vi "KE2606 Measuring.vi"(11 "VISA":refnum<visa-resource-name>) -> ()   [LabVIEW 2017]
doc: "This example shows how to configure the source and take a measurement."
uses:
  Channel.ctl
  Mesuring State.ctl
  <instrlib>/Keithley 2600 Series/Public/Channel.ctl
  <instrlib>/Keithley 2600 Series/Keithley 2600 Series.lvlib
panel:
  in  "Channel (Channel A)":T1
  in  "Voltage step, V":dbl=0.05
  in  "Voltage stop, V":dbl=2.0
  in  "Voltage start, V":dbl
  in  "Current limit, A":dbl=1.0
  in  "Channel":T2
  out "Measured current, A":dbl
  out "Sourced voltage, V":dbl
  out "I/V Curve":cluster{"X":dbl, "Y":dbl}[](graph) caption="XY Graph - Light"
  out "State":T3
  in  "Stop Button":bool
  in  "Start Button":bool
  in  "Exit Button":bool
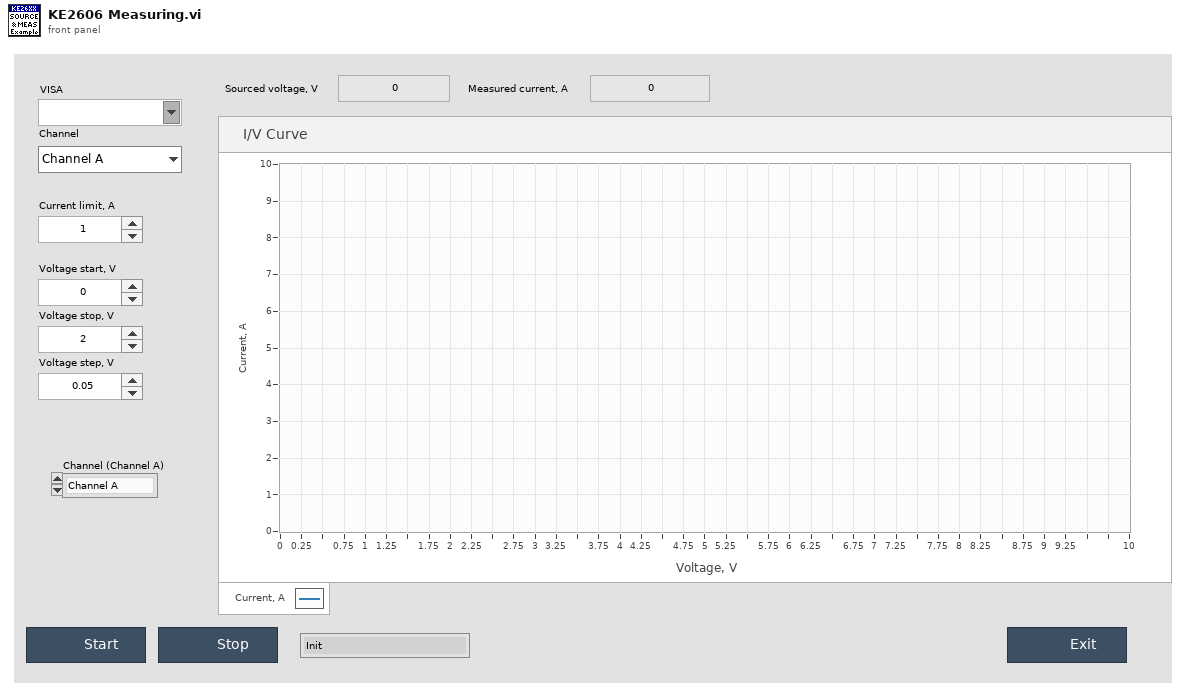
[diagram p1: front panel]
types:
  T1 = typedef "Keithley 2600 Series.lvlib/Channel.ctl" = enum32{"Channel A", "Channel B"}
  T2 = typedef "Channel.ctl" = enum32{"Channel A", "Channel B"}
  T3 = typedef "Mesuring State.ctl" = enum16{"Init", "Start", "Stop", "Nothing", "Exit"}
  T4 = enum32{"Current", "Voltage", "IV", "Resistance", "Power"}
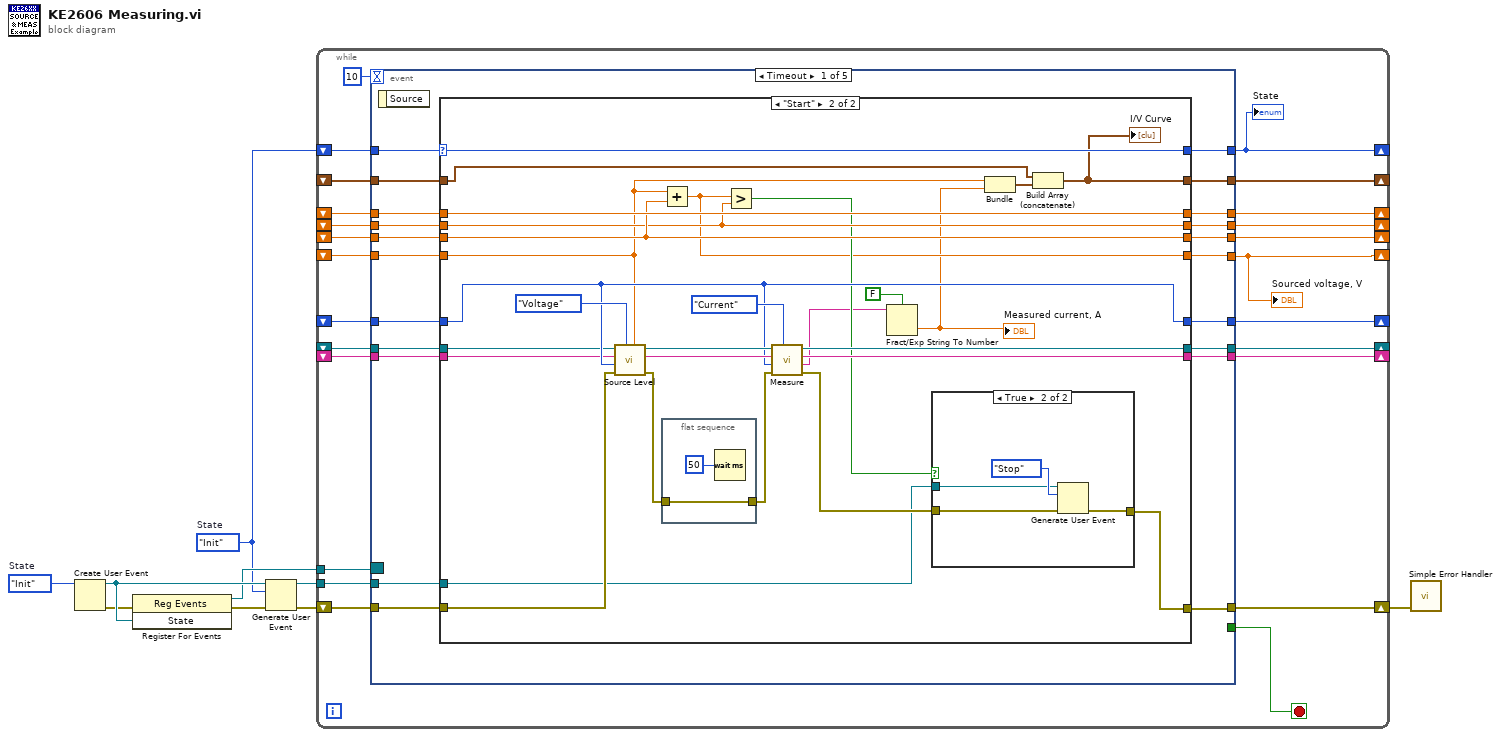
[diagram p0: block diagram]
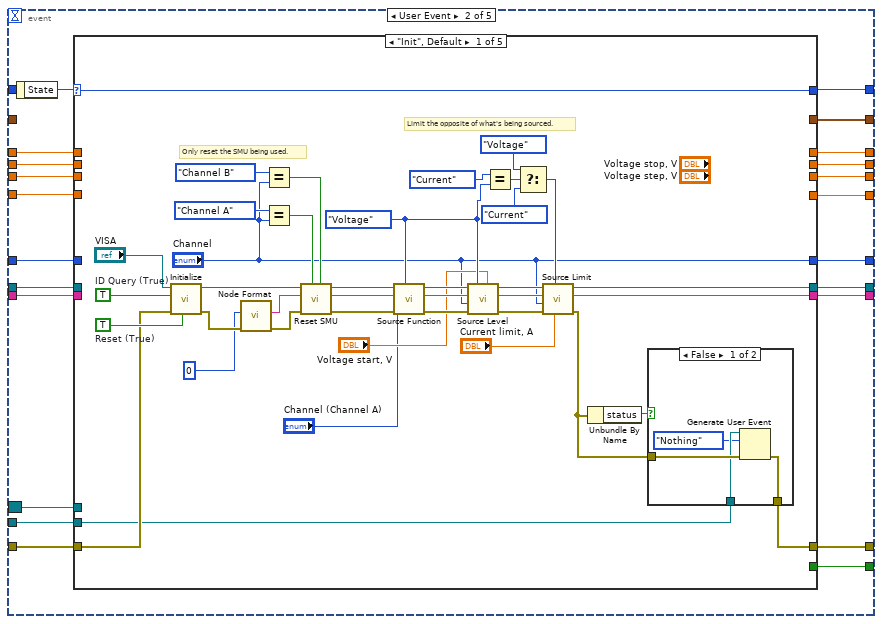
[diagram p4: hidden frame]
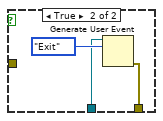
[diagram p5: hidden frame]
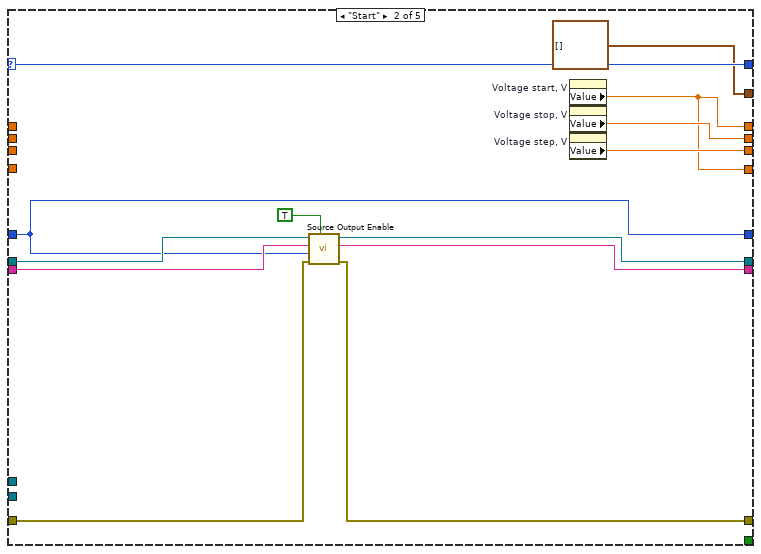
[diagram p6: hidden frame]
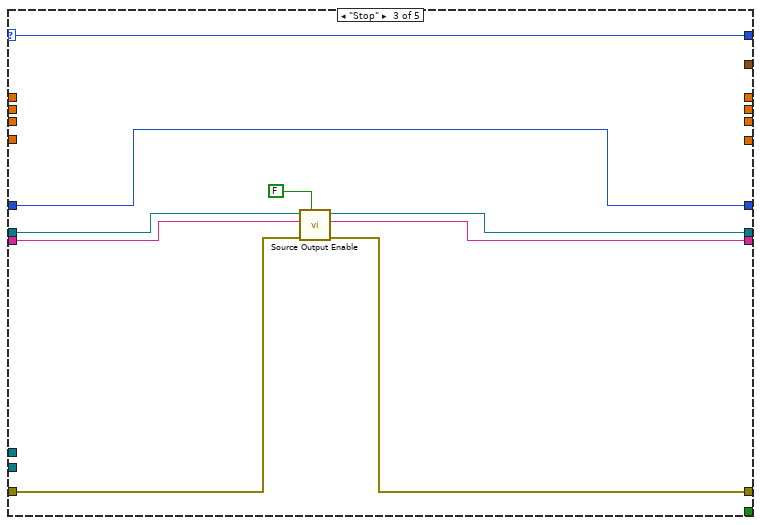
[diagram p7: hidden frame]
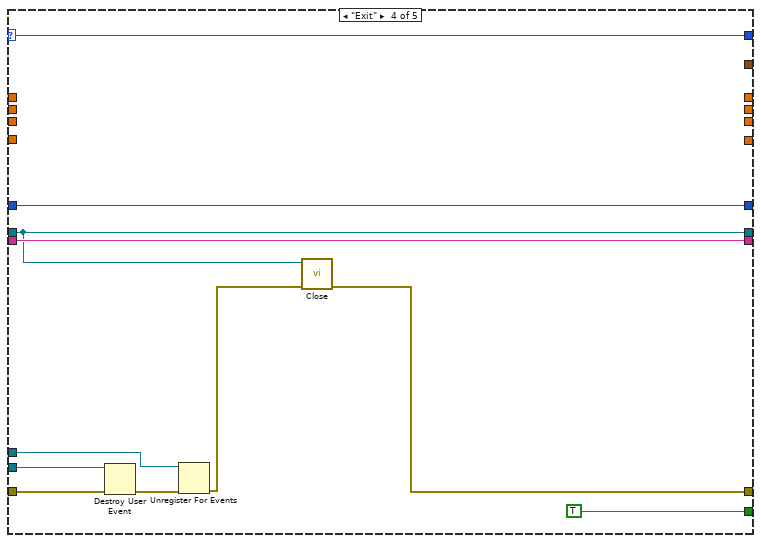
[diagram p8: hidden frame]
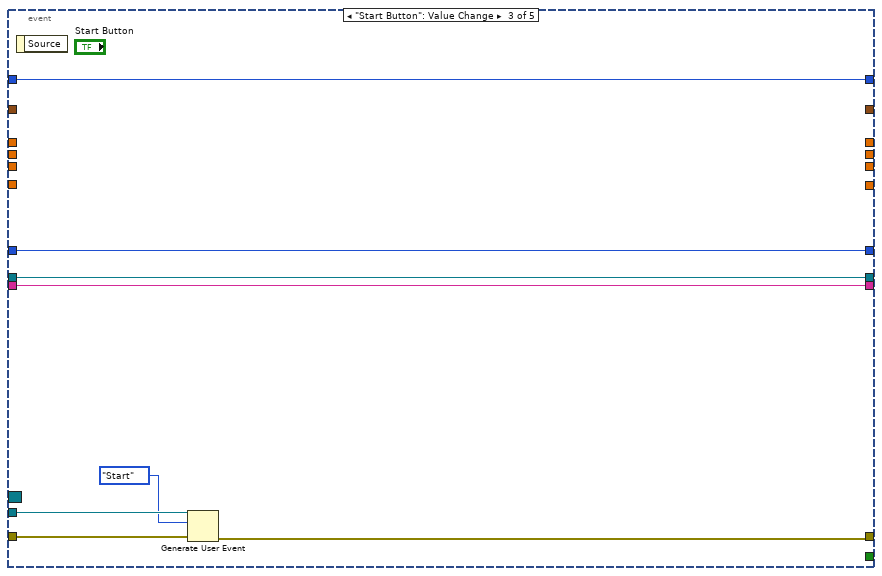
[diagram p10: hidden frame]
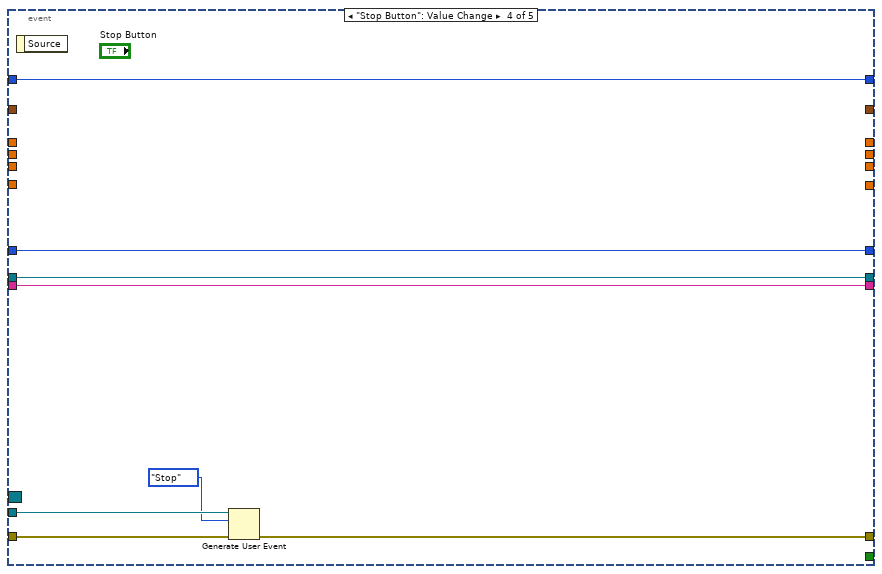
[diagram p11: hidden frame]
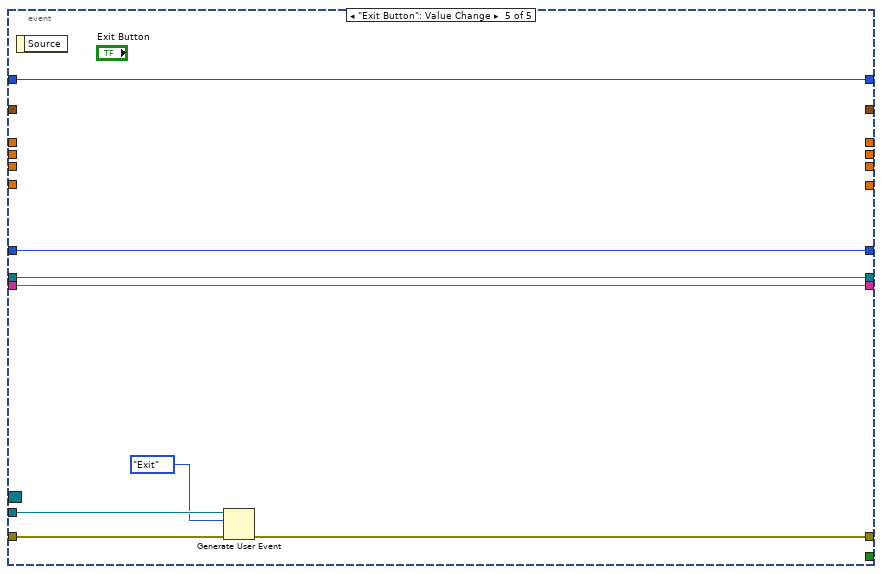
[diagram p12: hidden frame]
diagram:
  w1 = Mesuring_State."Init"  # State
  w3 = Mesuring_State."Init"  # State
  n1 = Create User Event(user event datatype=w3) -> (user event=w9:refnum<user-event>, error out=w7:errorcluster)  [unwired: 1 in]
  n2 = register-events(error in=w7, w9) -> (reference out=w6:refnum<event-registration>, error out=w8:errorcluster)  [unwired: 1 in]
  n3 = Generate User Event(user event=w9, event data cluster=w1, error in=w8) -> (user event out=w5:refnum<user-event>, error out=w4:errorcluster)  [unwired: 1 in]
  n4 = while {
    tunnel: w6 -> [w31]
    tunnel: w5 -> [w32]
    shift-right: [w30] -> w2
    shift-left: w4 -> [w33]
    shift-right: [w29] -> _
    shift-left: _ -> [w25]
    shift-right: [w28] -> _
    shift-left: _ -> [w24]
    shift-right: [w27] -> _
    shift-left: _ -> [w26]
    shift-right: [w23] -> _
    shift-left: w1 -> [w22]
    shift-right: [w19] -> _
    shift-left: _ -> [w15]
    shift-right: [w18] -> _
    shift-left: _ -> [w14]
    shift-right: [w17] -> _
    shift-left: _ -> [w16]
    shift-right: [w12] -> _
    shift-left: _ -> [w13]
    shift-right: [w11] -> _
    shift-left: _ -> [w10]
    stop <- w20 stop-if-true
    n5 = event shown="[0] Timeout" {
      selector: w31 -> [_ w110 _ _ _]
      dyn-events: _ -> [_ _ _ _ _]
      timeout: 10 -> [_ _ _ _ _]
      tunnel: w33 -> [w46 w119 w208 w217 w224]
      tunnel: w32 -> [w36 w120 w209 w215 w225]
      tunnel: [w45 w118 w207 w216 w222] -> w30
      tunnel: [w49 w117 w211 w219 w227] -> w29
      tunnel: [w47 w116 w210 w218 w226] -> w28
      tunnel: [w51 w115 w212 w220 w228] -> w27
      tunnel: w26 -> [w52 w114 w212 w220 w228]
      tunnel: w25 -> [w50 w113 w211 w219 w227]
      tunnel: w24 -> [w48 w112 w210 w218 w226]
      tunnel: [w53 w111 w213 w221 w229] -> w23
      tunnel: w22 -> [w54 _ w213 w221 w229]
      tunnel: [_ w109 _ _ _] -> w20
      tunnel: [w39 w108 _ _ _] -> w19
      tunnel: [w38 w107 _ _ _] -> w18
      tunnel: [w43 w106 _ _ _] -> w17
      tunnel: w16 -> [w44 w105 _ _ _]
      tunnel: w15 -> [w42 w104 _ _ _]
      tunnel: w14 -> [w41 w103 _ _ _]
      tunnel: [w37 w102 _ _ _] -> w12
      tunnel: w13 -> [w40 w101 _ _ _]
      tunnel: [w35 w100 _ _ _] -> w11
      tunnel: w10 -> [w34 _ _ _ _]
      event Timeout {
        n6 = event-data() -> ()  [unwired: 1 in, 1 out]
        n7 = case shown="\"Start\"" w54 {
          selector: w54 -> [w64 w92]
          tunnel: [w64 w92] -> w53
          tunnel: [w63 w85] -> w51
          tunnel: w52 -> [w63 w85]
          tunnel: w50 -> [w62 w84]
          tunnel: [w62 w89] -> w49
          tunnel: w48 -> [w61 w83]
          tunnel: [w61 w90] -> w47
          tunnel: w46 -> [w60 w82]
          tunnel: [w60 w76] -> w45
          tunnel: [w59 w81] -> w43
          tunnel: w44 -> [w59 w81]
          tunnel: w42 -> [w58 w79]
          tunnel: w41 -> [w57 w80]
          tunnel: w40 -> [w56 w71]
          tunnel: [w58 w79] -> w39
          tunnel: [w57 w80] -> w38
          tunnel: [w56 w75] -> w37
          tunnel: w36 -> [_ w74]
          tunnel: [w55 w67] -> w35
          tunnel: w34 -> [w55 w68]
          frame Default {
          }
          frame "Start" {
            n8 = call <instrlib>:"Source Level.vi"("Level (0.000)"=w71, "Function (Current)"=enum32{"Current", "Voltage"}."Voltage", "error in (no error)"=w82, "Channel (Channel A)"=w85, "Node In"=w83, "VISA resource name"=w84) -> ("error out"=w66:errorcluster, "Node Out"=w87:string, "VISA resource name out"=w86:refnum<visa-resource-name>)  [unwired: 3 out]
            n9 = Add(x=w71, y=w80) -> (x+y=w75:dbl)
            n10 = flat-sequence {
              tunnel: w66 -> [w94]
              tunnel: [w94] -> w65
              frame #0 {
                n11 = Wait (ms)(milliseconds to wait=u32 50) -> ()  [unwired: 1 out]
              }
            }
            n12 = Greater?(x=w75, y=w79) -> (0:w78:bool)
            n13 = call <instrlib>:"Measure.vi"("Function (Current)"=T4."Current", "error in (no error)"=w65, "Channel (Channel A)"=w85, "Node In"=w87, "VISA resource name"=w86) -> ("error out"=w77:errorcluster, "Output"=w73:string, "Node Out"=w90:string, "VISA resource name out"=w89:refnum<visa-resource-name>)  [unwired: 2 in, 1 out]
            n14 = Fract/Exp String To Number(use system decimal point (T)=FALSE, string=w73) -> (number=w70:dbl)  [unwired: 2 in, 1 out]
            "Measured current, A" <- w70
            n15 = case shown="True" w78 {
              tunnel: w77 -> [w95 w98]
              tunnel: [w95 w97] -> w76
              tunnel: w74 -> [_ w96]
              frame False {
              }
              frame True {
                n16 = Generate User Event(user event=w96, event data cluster=Mesuring_State."Stop" ("event data"), error in=w98) -> (error out=w97:errorcluster)  [unwired: 1 in, 1 out]
              }
            }
            n17 = Bundle("Value"=w71, w70) -> (w69:cluster{"Value":dbl, dbl})  [unwired: 1 in]
            n18 = Build Array (concatenate)(w68, w69) -> (w67:cluster{"Value":dbl, "Y":dbl}[])
            "I/V Curve" <- w67
          }
        }
      }
      event User Event {
        n19 = event-data() -> ("State"=w121:T3)  [unwired: 1 in]
        n20 = case shown="\"Init\", Default" w121 {
          selector: w121 -> [w129 w172 w181 w196 w202]
          tunnel: w120 -> [w125 _ _ w199 _]
          tunnel: w119 -> [w132 w177 w183 w200 w201]
          tunnel: [w126 w176 w182 w190 w201] -> w118
          tunnel: [w131 w174 w185 w192 w204] -> w117
          tunnel: [w130 w173 w186 w194 w203] -> w116
          tunnel: ["Channel" w175 w184 w195 w205] -> w115
          tunnel: w114 -> [_ w175 w184 w195 w205]
          tunnel: w113 -> [_ w179 w188 w192 w204]
          tunnel: w112 -> [_ w178 w187 w194 w203]
          tunnel: [w129 w172 w181 w196 w202] -> w111
          tunnel: w110 -> [_ _ _ w197 _]
          tunnel: [_ _ _ TRUE _] -> w109
          tunnel: [_ w171 _ _ _] -> w108
          tunnel: [_ w170 _ _ _] -> w107
          tunnel: [_ w169 _ _ _] -> w106
          tunnel: w105 -> [_ _ _ _ _]
          tunnel: w104 -> [_ _ _ _ _]
          tunnel: w103 -> [_ _ _ _ _]
          tunnel: [_ w169 _ _ _] -> w102
          tunnel: w101 -> [_ _ _ _ _]
          tunnel: [_ cluster{"X":dbl, "Y":dbl}[] [] ("I/V Curve") _ _ _] -> w100
          frame "Init", Default {
            w140 = enum32{"Current", "Voltage"}."Voltage" ("Source Function (Current)")
            w134 = TRUE  # Reset (True)
            w133 = TRUE  # ID Query (True)
            # "Limit the opposite of what's being sourced."
            # "Only reset the SMU being used."
            n21 = call <instrlib>:"Initialize.vi"("Reset (True)"=w134, "error in (no error)"=w132, "ID Query (True)"=w133, "VISA resource name"="VISA") -> ("error out"=w158:errorcluster, "VISA resource name out"=w143:refnum<visa-resource-name>)  [unwired: 2 in, 4 out]
            n22 = call <instrlib>:"Node Format.vi"("error in"=w158, "Node (0-64)"=i8 0) -> ("error out"=w159:errorcluster, "Formatted Node"=w157:string)  [unwired: 8 out]
            n23 = Equal?(x=enum32{"Channel A", "Channel B"}."Channel B", y="Channel") -> (x = y?=w145:bool)
            n24 = Equal?(x=enum32{"Channel A", "Channel B"}."Channel A", y="Channel") -> (x = y?=w144:bool)
            n25 = call <instrlib>:"Reset SMU.vi"("SMU B (No)"=w145, "SMU A (No)"=w144, "error in (no error)"=w159, "Node In"=w157, "VISA resource name"=w143) -> ("error out"=w146:errorcluster, "Node Out"=w148:string, "VISA resource name out"=w147:refnum<visa-resource-name>)  [unwired: 4 out]
            n26 = call <instrlib>:"Source Function.vi"("Function (Current)"=w140, "error in (no error)"=w146, "Channel (Channel A)"="Channel (Channel A)", "Node In"=w148, "VISA resource name"=w147) -> ("error out"=w151:errorcluster, "Node Out"=w149:string, "VISA resource name out"=w150:refnum<visa-resource-name>)  [unwired: 4 out]
            n27 = call <instrlib>:"Source Level.vi"("Level (0.000)"="Voltage start, V", "Function (Current)"=w140, "error in (no error)"=w151, "Channel (Channel A)"="Channel", "Node In"=w149, "VISA resource name"=w150) -> ("error out"=w152:errorcluster, "Node Out"=w154:string, "VISA resource name out"=w153:refnum<visa-resource-name>)  [unwired: 3 out]
            n28 = Equal?(x=enum32{"Current", "Voltage"}."Current", y=w140) -> (x = y?=w155:bool)
            n29 = Select(t=enum32{"Current", "Voltage"}."Voltage" ("x"), s=w155, f=enum32{"Current", "Voltage"}."Current") -> (s? t:f=w156:enum32{"Current", "Voltage"})
            n30 = call <instrlib>:"Source Limit.vi"("Limit (0.000)"="Current limit, A", "Function (Current)"=w156, "error in (no error)"=w152, "Channel (Channel A)"="Channel", "Node In"=w154, "VISA resource name"=w153) -> ("error out"=w127:errorcluster, "Node Out"=w130:string, "VISA resource name out"=w131:refnum<visa-resource-name>)  [unwired: 3 out]
            n31 = Unbundle By Name(w127) -> ("status"=w128:bool)
            n32 = case shown="False" w128 {
              tunnel: w127 -> [w164 _]
              tunnel: [w163 w165] -> w126
              tunnel: w125 -> [w162 w166]
              frame False {
                n33 = Generate User Event(user event=w162, event data cluster=Mesuring_State."Nothing" ("event data"), error in=w164) -> (error out=w163:errorcluster)  [unwired: 1 in, 1 out]
              }
              frame True {
                n34 = Generate User Event(user event=w166, event data cluster=Mesuring_State."Exit" ("event data")) -> (error out=w165:errorcluster)  [unwired: 2 in, 1 out]
              }
            }
          }
          frame "Start" {
            n35 = call <instrlib>:"Source Output Enable.vi"("Output (Off)"=TRUE, "error in (no error)"=w177, "Channel (Channel A)"=w175, "Node In"=w178, "VISA resource name"=w179) -> ("error out"=w176:errorcluster, "Node Out"=w173:string, "VISA resource name out"=w174:refnum<visa-resource-name>)  [unwired: 4 out]
            n36 = property on="Voltage start, V" class="DigNum (strict)"() -> ("Value"=w169:dbl)  [unwired: 2 in, 2 out]
            n37 = property on="Voltage stop, V" class="DigNum (strict)"() -> ("Value"=w171:dbl)  [unwired: 2 in, 2 out]
            n38 = property on="Voltage step, V" class="DigNum (strict)"() -> ("Value"=w170:dbl)  [unwired: 2 in, 2 out]
          }
          frame "Stop" {
            n39 = call <instrlib>:"Source Output Enable.vi"("Output (Off)"=FALSE, "error in (no error)"=w183, "Node In"=w187, "VISA resource name"=w188) -> ("error out"=w182:errorcluster, "Node Out"=w186:string, "VISA resource name out"=w185:refnum<visa-resource-name>)  [unwired: 1 in, 4 out]
          }
          frame "Exit" {
            n40 = Destroy User Event(user event=w199, error in=w200) -> (error out=w198:errorcluster)
            n41 = Unregister For Events(event registration refnum=w197, error in=w198) -> (error out=w191:errorcluster)
            n42 = call <instrlib>:"Close.vi"("error in (no error)"=w191, "VISA resource name"=w192) -> ("error out"=w190:errorcluster)  [unwired: 9 out]
          }
          frame "Nothing" {
          }
        }
      }
      event "Start Button": Value Change {
        n43 = event-data() -> ()  [unwired: 1 in, 1 out]
        n44 = Generate User Event(user event=w209, event data cluster=Mesuring_State."Start" ("event data"), error in=w208) -> (error out=w207:errorcluster)  [unwired: 1 in, 1 out]
      }
      event "Stop Button": Value Change {
        n45 = event-data() -> ()  [unwired: 1 in, 1 out]
        n46 = Generate User Event(user event=w215, event data cluster=Mesuring_State."Stop" ("event data"), error in=w217) -> (error out=w216:errorcluster)  [unwired: 1 in, 1 out]
      }
      event "Exit Button": Value Change {
        n47 = event-data() -> ()  [unwired: 1 in, 1 out]
        n48 = Generate User Event(user event=w225, event data cluster=Mesuring_State."Exit" ("event data"), error in=w224) -> (error out=w222:errorcluster)  [unwired: 1 in, 1 out]
      }
    }
    "State" <- w23
    "Sourced voltage, V" <- w12
  }
  n49 = call <vilib>:"Simple Error Handler.vi"("error in (no error)"=w2) -> ()  [unwired: 4 in, 5 out]
